vi "Launch_Queue_Comm_FGV.vi"(8 "error in (no error)":errorcluster, 10 "Enum":T1, 11 "queue in":refnum<queue>) -> (0 "error Out":errorcluster, 3 "queue Out":refnum<queue>)   [LabVIEW 2024, in "LaunchTest.lvlib"]
doc: "This VI\n-----------------------------------\nQueue_Comm_FGV\n-----------------------------------\n-Craetes a FG varaibale for queue reference"
uses:
  LaunchTest.lvlib
  support/Message Queue/Launch_Message Cluster.ctl
  support/Message Queue/Launch_Message Queue.lvlib
  PrivateControls/Launch_FGV_Queue_Control.ctl
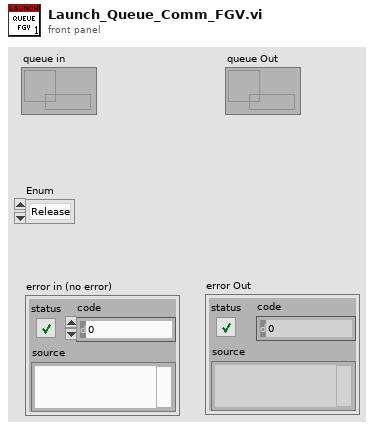
[diagram p1: front panel]
types:
  T1 = typedef "LaunchTest.lvlib/Launch_FGV_Queue_Control.ctl" = enum16{"Release", "Get", "Set", "Flush"}
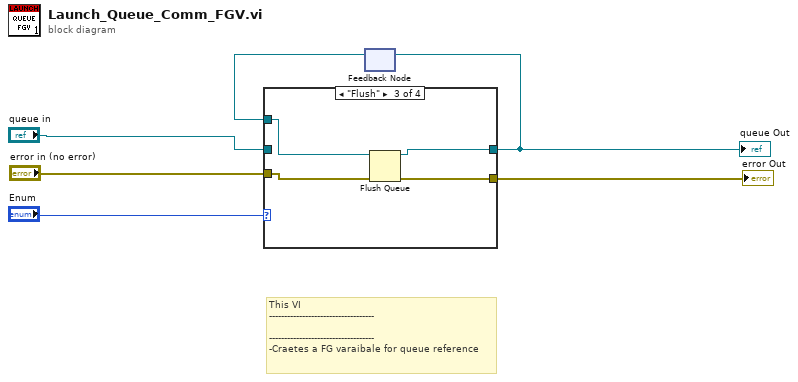
[diagram p0: block diagram]
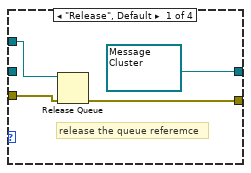
[diagram p2: hidden frame]
diagram:
  # "This VI\n-----------------------------------\n\n-----------------------------------\n-Craetes a FG varaibale for queue reference"
  n1 = feedback #1() -> (w5:refnum<queue>)  [unwired: 1 in]
  n2 = case shown="\"Flush\"" "Enum" {
    tunnel: "queue in" -> [_ _ _ w18]
    tunnel: [refnum<queue> refnum ("queue out") w12 w13 w18] -> w1
    tunnel: w5 -> [w7 w12 w14 _]
    tunnel: "error in (no error)" -> [w10 w11 w16 w17]
    tunnel: [w9 w11 w15 w17] -> w3
    frame "Release", Default {
      # "release the queue referemce"
      n3 = Release Queue(queue=w7, error in (no error)=w10) -> (error out=w9:errorcluster)  [unwired: 1 in, 2 out]
    }
    frame "Get" {
      # "get  the queue reference in FGV"
    }
    frame "Flush" {
      n4 = Flush Queue(queue=w14, error in (no error)=w16) -> (queue out=w13:refnum<queue>, error out=w15:errorcluster)  [unwired: 1 out]
    }
    frame "Set" {
      # "set the queue reference in FGV"
    }
  }
  "error Out" <- w3
  "queue Out" <- w1
  n5 = feedback-in #1(w1) -> ()
